vi "Override State Pointer.vi"(8 "error in (no error)":errorcluster, 10 "new state pointer":refnum<class "Pointer.lvclass">, 11 "Thread in":refnum<class "Thread.lvclass">) -> (0 "error out":errorcluster, 3 "Thread out":refnum<class "Thread.lvclass">)   [LabVIEW 2020, in "DSF Core.lvlib" / "Thread.lvclass"]
uses:
  Thread.lvclass
  <vilib>/NI/Memory Manager/Classes/Pointer/Pointer.lvclass
  Thread.lvclass/Thread.ctl
  <vilib>/NI/Memory Manager/Classes/Pointer/Pointer.lvclass/Pointer.ctl
  <vilib>/NI/Memory Manager/Classes/Pointer/Get Address.vi
  <vilib>/NI/Memory Manager/Classes/Pointer/Get Internal.vi
  <vilib>/NI/Memory Manager/Classes/Pointer/Errors.vi
  <vilib>/NI/Memory Manager/Classes/Pointer/Zone.vi
  <vilib>/NI/Memory Manager/Classes/Pointer/Set Address.vi
  <vilib>/NI/Memory Manager/Classes/Pointer/Set Size.vi
  <vilib>/NI/Memory Manager/Classes/Pointer/Set Internal.vi
  <vilib>/NI/Memory Manager/Classes/Pointer/Check Null Pointer.vi
  <vilib>/NI/Memory Manager/Classes/Pointer/Create Error.vi
  <vilib>/NI/Memory Manager/Classes/Pointer/Null Pointer.vi
  <vilib>/NI/Memory Manager/VIs/New Error Cluster.vi
  <vilib>/NI/Memory Manager/VIs/New Error Cluster (512B).vi
  <vilib>/NI/Memory Manager/VIs/Set Error Status.vi
  <vilib>/NI/Memory Manager/VIs/Set Error Code.vi
  <vilib>/NI/Memory Manager/VIs/Set Error Source.vi
  <vilib>/NI/Memory Manager/Constants/Constants.vi
  <vilib>/NI/Memory Manager/Constants/Library Name.vi
  <vilib>/NI/Memory Manager/Classes/Pointer/Pointer Error Info.vi
  <vilib>/NI/Memory Manager/VIs/Write String to Source.vi
  <vilib>/NI/Memory Manager/Constants/Pointer Class Name.vi
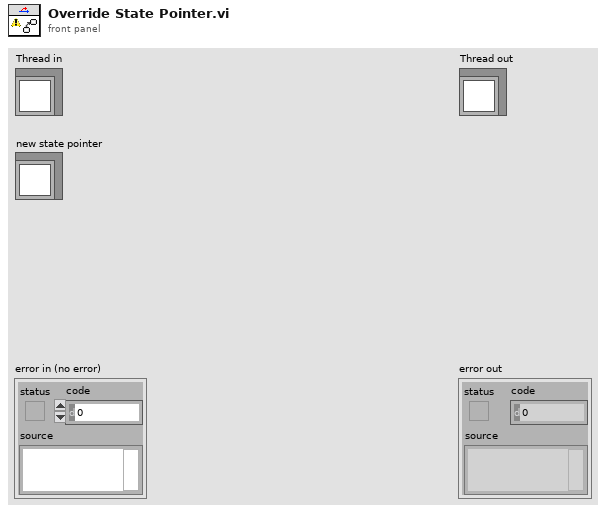
[diagram p1: front panel]
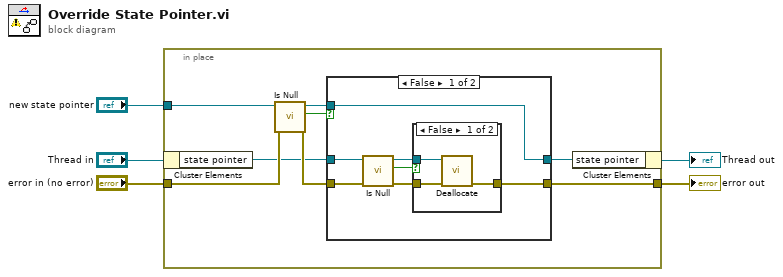
[diagram p0: block diagram]
diagram:
  n1 = in-place {
    in-place-border: "new state pointer" -> [w13]
    in-place-border: "error in (no error)" -> [w11]
    in-place-border: [w6] -> w1
    n2 = in-place-cluster #1("Thread in") -> ("state pointer"=w9:refnum<class "Pointer.lvclass">)
    n3 = call <vilib>:"Is Null.vi"("error in (no error)"=w11, "Pointer in"=w13) -> ("error out"=w10:errorcluster, "null?"=w12:bool, "Pointer out"=w8:refnum<class "Pointer.lvclass">)  [unwired: 7 in]
    n4 = case shown="False" w12 {
      tunnel: w9 -> [w20 w26]
      tunnel: w10 -> [w16 w25]
      tunnel: w8 -> [w14 _]
      tunnel: [w14 w26] -> w7
      tunnel: [w15 w25] -> w6
      frame False {
        n5 = call <vilib>:"Is Null.vi"("error in (no error)"=w16, "Pointer in"=w20) -> ("error out"=w17:errorcluster, "null?"=w18:bool, "Pointer out"=w19:refnum<class "Pointer.lvclass">)  [unwired: 7 in]
        n6 = case shown="False" w18 {
          tunnel: w19 -> [w23 _]
          tunnel: w17 -> [w22 w24]
          tunnel: [w21 w24] -> w15
          frame False {
            n7 = call <vilib>:"Deallocate.vi"("error in (no error)"=w22, "Pointer"=w23) -> ("error out"=w21:errorcluster)  [unwired: 8 in, 1 out]
          }
          frame True {
          }
        }
      }
      frame True {
      }
    }
    n8 = in-place-cluster #1("state pointer"=w7) -> (→"Thread out":refnum<class "Thread.lvclass">)
  }
  "error out" <- w1
